vi "ecg_ncs_v2.vi"() -> ()   [LabVIEW 2016]
uses:
  <instrlib>/niUSRP/niUSRP Timestamp.ctl
  C:/Program Files/National Instruments/LabVIEW 2016/examples/Instrument IO/Serial/support/Serial - Settings.ctl
  State.ctl
  <vilib>/Instr/_visa.llb/VISA Configure Serial Port (Instr).vi
  <instrlib>/niUSRP/niUSRP Write Tx Data (2D CDB).vi
  <instrlib>/niUSRP/niUSRP Fetch Rx Data (2D CDB).vi
panel:
  out "ECGsample":i16
  out "PhNcs":dbl
  out "AmpNcs":dbl
  out "AmpNcsDS":dbl
  out "PhNcsDS":dbl
  in  "File Name":string="Test"
  in  "Path":path=path "D:/Research/SummerFall17Spring18/CnC/NCS/EcgNcsCorrelation/Labview Codes/ECG_NCS"
  out "error IO 2":errorcluster={"status"=FALSE, "code"=-1074118647, "source"=""}
  in  "Serial Settings":T1={"baud rate"=57600, "data bits"=8, "parity"=enum."None", "stop bits"=10, "flow control"=0} {"flow control" items=["None"=0, "XON/XOFF"=1, "RTS/CTS"=2, "DTR/DSR"=4]; "stop bits" items=["1.0"=10, "1.5"=15, "2.0"=20]; "data bits" min=5 max=8 step=1; "baud rate" items=["75"=75, "110"=110, "134"=134, "150"=150, "300"=300, "600"=600, "1200"=1200, "1800"=1800, "2400"=2400, "4800"=4800, "7200"=7200, "9600"=9600, "14400"=14400, "19200"=19200, "28800"=28800, "38400"=38400, "56000"=56000, "57600"=57600, "115200"=115200, "128000"=128000, "230400"=230400]}
  in  "VISA resource name":refnum<visa-resource-name>="bmd101"
  out "Packets Recieved":i32
  out "ECG":i16(graph)
  in  "byte count":u32=1
  out "Coerced Rx IQ Rate":dbl
  in  "Sampling Rate":i32=500
  out "Gain":dbl=-15.0
  out "Bandwidth":dbl=56000000.0
  out "Coerced Carrier Frequency":dbl=2000000000.0 format="%#.17g"
  out "Coerced Tx IQ rate":dbl=1000000.0
  out "error IO":errorcluster={"status"=FALSE, "code"=-1074118647, "source"=""}
  in  "Rx Number of Samples":i32=20000
  in  "Tab Control 2":enum32{"NI-294x/295x", "NI-2900/2901"}(tab)=enum."NI-2900/2901"
  in  "Rx carrier frequency [Hz]":dbl=2000000000.0 format="%#_6p"
  in  "Tx carrier frequency [Hz]":dbl=1000000000.0 format="%#_6p"
  in  "Start Trigger Time":T2={"whole seconds"=1, "fractional seconds"=0.0}
  in  "Tab Control":T3(tab)
  out "NCS tag Amp":dbl[](graph)=[0.011967714738528729, 0.012021355192189592, 0.012015275039596582, 0.011969166030167903, 0.011958890166168242, 0.012007893820858737, 0.012022893722444085, 0.011978222225113794, 0.011969989939463181, 0.012003099640895068]
  out "NCS tag Phase":dbl[](graph)=[0.011967714738528729, 0.012021355192189592, 0.012015275039596582, 0.011969166030167903, 0.011958890166168242, 0.012007893820858737, 0.012022893722444085, 0.011978222225113794, 0.011969989939463181, 0.012003099640895068]
  out "Tag Amp":dbl[](graph)
  out "Tag Phase":dbl[](graph)
  out "Tx Waveform Graph":waveform(dbl)[](graph)
  in  "Stop":bool
  in  "Channel 0\nTone Amplitude":dbl=0.707 step=0.05 format="%#.6g"
  in  "Channel 0 \nTone Frequency":dbl=5000.0 format="%#_6p"
  in  "Tx Waveform Size":dbl=2000.0
  in  "Device Name":refnum<k15>="MyB200"
  in  "Tx Gain":dbl=28.0 format="%#_6f"
  in  "Tx IQ Rate":dbl=1000000.0 format="%#_6p"
  in  "Rx Gain":dbl=32.0 format="%#_6f"
  in  "Rx IQ Rate":dbl=1000000.0 format="%#_6p"
  # "Rx Settings"
  # "Tx Settings"
  # "Note that on the NI-2900 and NI-2901, both Rx channels share an LO and both Tx channels share an LO. However, on the NI-294x/295x devices, Rx and Tx of channel 0 share an LO and Rx and Tx of channel 1 share an LO."
  # "Rx: Number of samples should be 1e6/512 in one loop."
  # "This Tx graph should always have end and start tied up since this is being sent in a loop continuously. Otherwise phase jumps will be noticed."
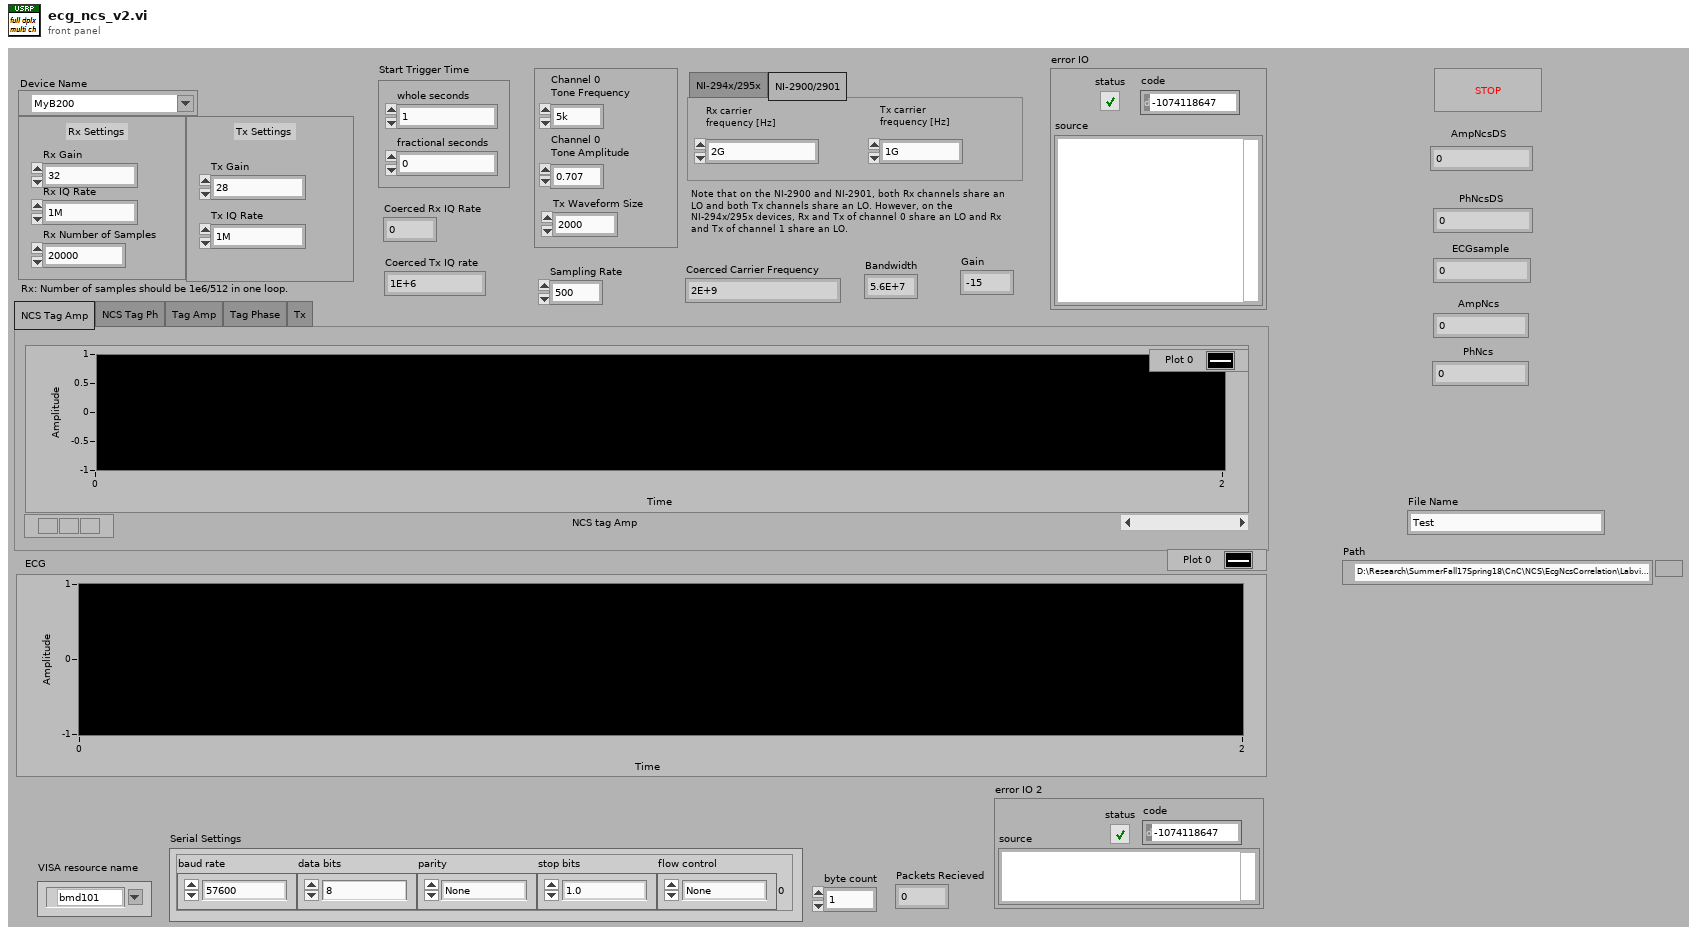
[diagram p1: front panel]
types:
  T1 = typedef "Serial - Settings.ctl" = cluster{"baud rate":u32, "data bits":u16, "parity":enum16{"None", "Odd", "Even", "Mark", "Space"}, "stop bits":u16, "flow control":u16}
  T2 = typedef "niUSRP Timestamp.ctl" = cluster{"whole seconds":u64, "fractional seconds":dbl}
  T3 = enum32{"NCS Tag Amp", "NCS Tag Ph", "Tag Amp", "Tag Phase", "Tx"}
  T4 = typedef "State.ctl" = enum16{"Initialize", "get byte", "check", "packet received", "packet approved"}
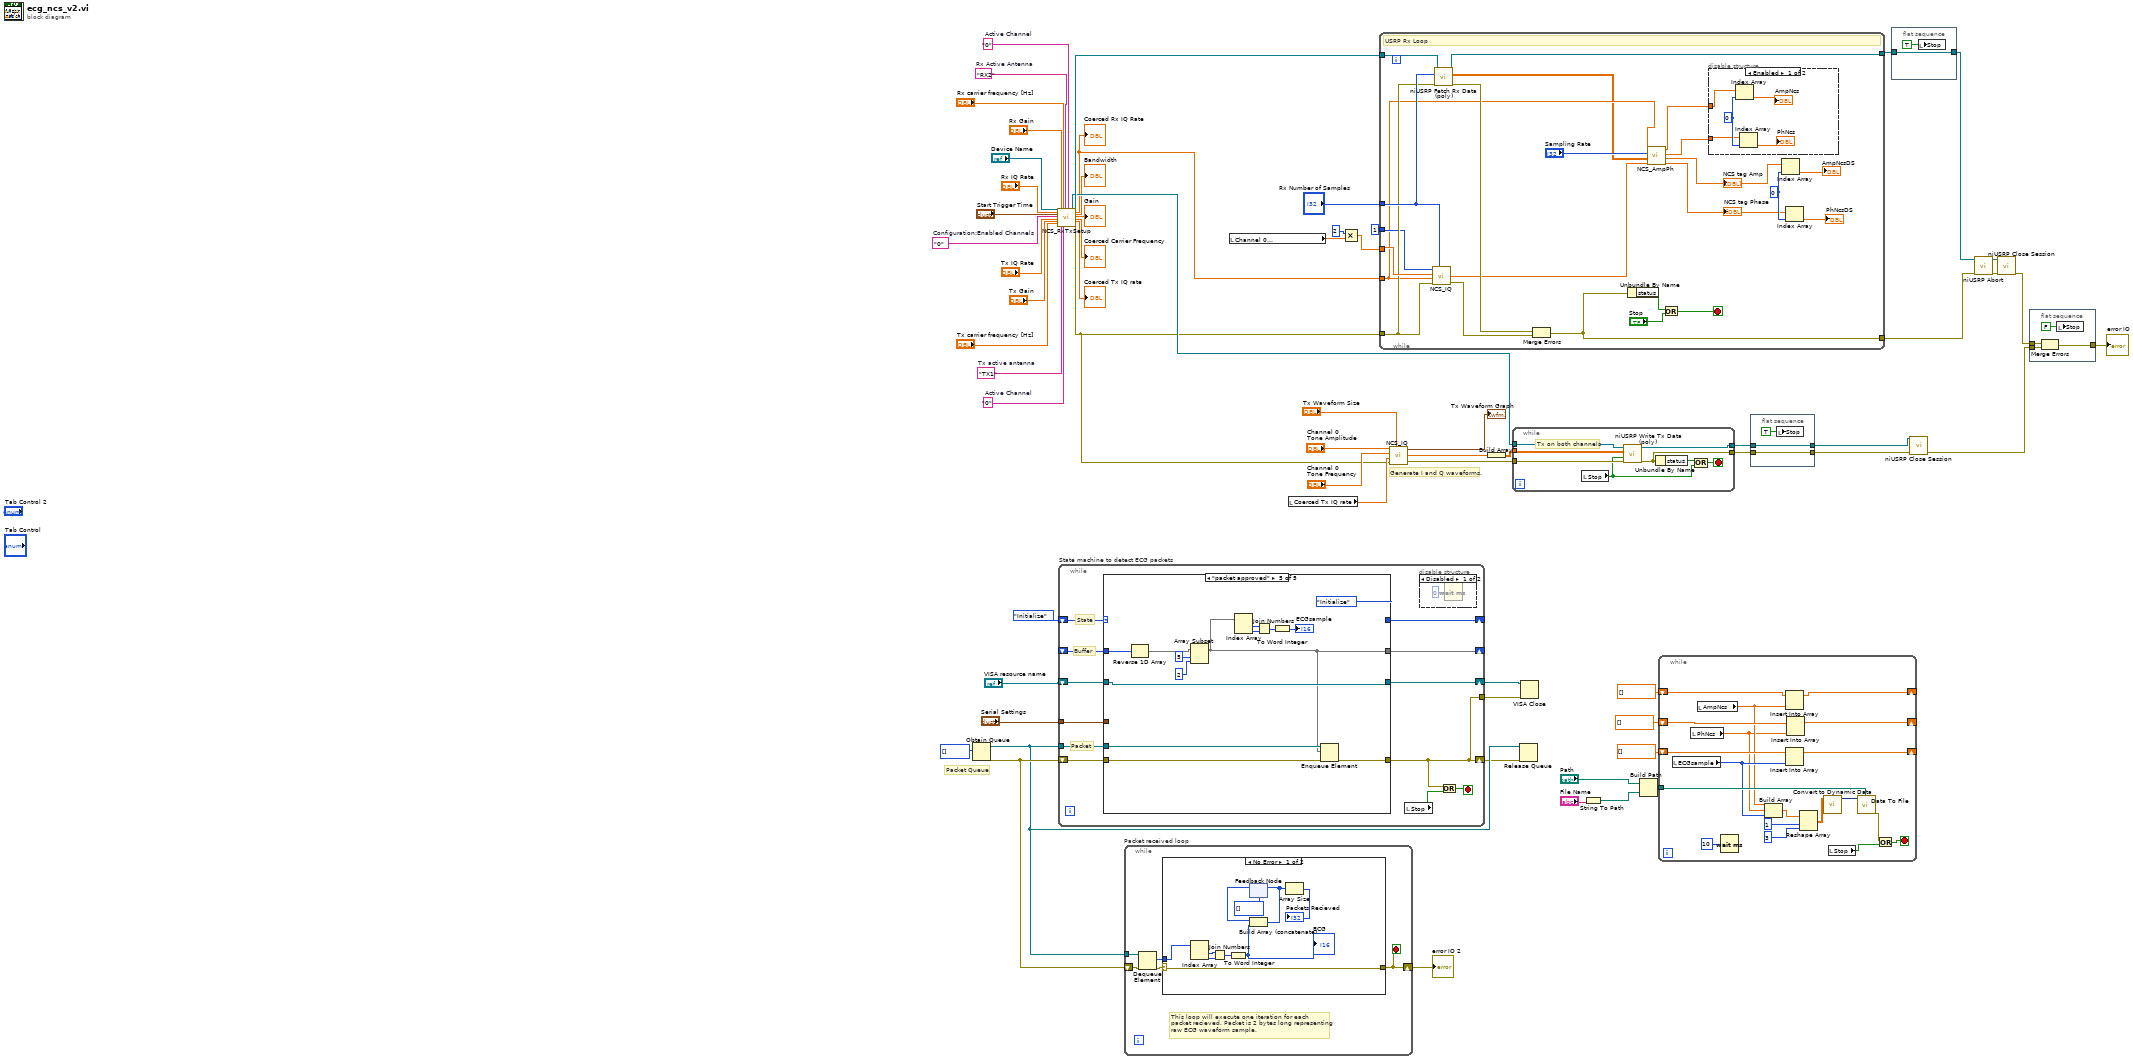
[diagram p0: block diagram]
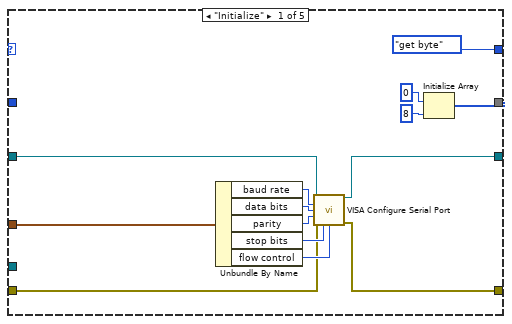
[diagram p4: hidden frame]
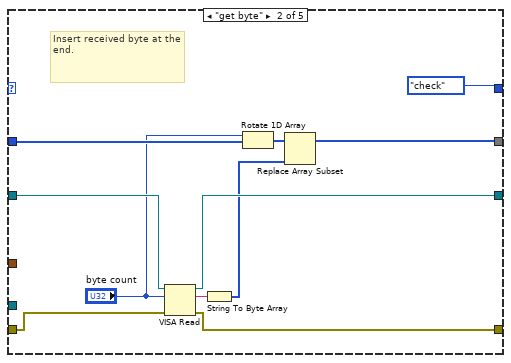
[diagram p5: hidden frame]
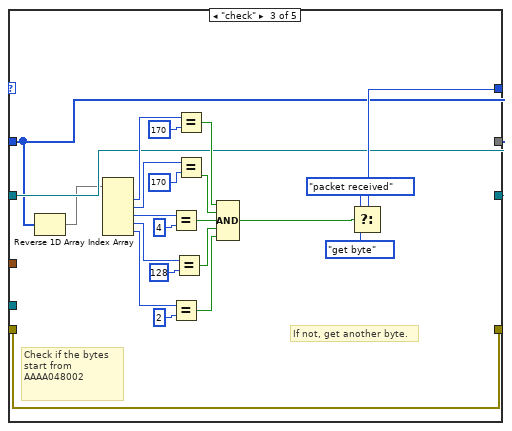
[diagram p6: hidden frame]
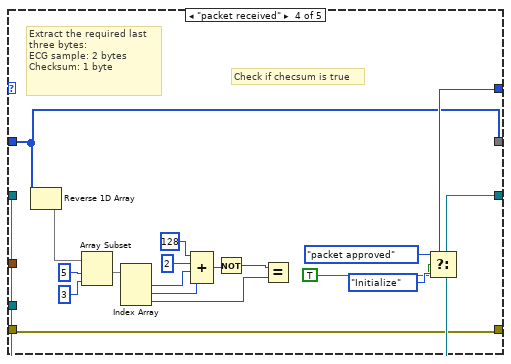
[diagram p7: hidden frame]
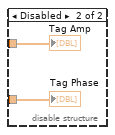
[diagram p8: hidden frame]
diagram:
  w19 = "0"  # Active Channel
  w20 = "0"  # Active Channel
  w55 = "RX2"  # Rx Active Antenna
  w51 = "TX1"  # Tx active antenna
  w37 = "0"  # Configuration:Enabled Channels
  # "Packet Queue"
  # "Generate I and Q waveforms."
  n1 = Obtain Queue(element data type=u8[] []) -> (queue out=w14:refnum<queue>, error out=w15:errorcluster)  [unwired: 4 in, 1 out]
  n2 = call "NCS_RxTxSetup.vi"("IVI Refnum in"="Device Name", "Rx IQ Rate"="Rx IQ Rate", "Start Trigger Time"="Start Trigger Time", "Configuration:Enabled Channels"=w37, "Tx IQ Rate"="Tx IQ Rate", "Tx Gain"="Tx Gain", "Tx carrier frequency [Hz]"="Tx carrier frequency [Hz]", "Rx Gain"="Rx Gain", "Tx active antenna"=w51, "Rx carrier frequency [Hz]"="Rx carrier frequency [Hz]", "Active Channel"=w19, "Rx Active Antenna"=w55, "Active Channel 2"=w20) -> ("session handle out"=w62:refnum<k15>, "IVI Refnum out"=w63:refnum<k15>, "Coerced Rx IQ Rate"=w18:dbl, "Bandwidth"=→"Bandwidth":dbl, "Gain"=→"Gain":dbl, "Carrier Frequency"=→"Coerced Carrier Frequency":dbl, "IQ Rate 2"=→"Coerced Tx IQ rate":dbl, "error out"=w30:errorcluster)  [unwired: 7 in]
  "Coerced Rx IQ Rate" <- w18
  n3 = while "State machine to detect ECG packets" {
    shift-right: [w66] -> w9
    shift-left: w15 -> [w72]
    shift-right: [w75] -> _
    shift-left: State."Initialize" ("State") -> [w74]
    shift-right: [w71] -> _
    shift-left: _ -> [w73]
    tunnel: w14 -> [w70]
    shift-right: [w69] -> w10
    shift-left: "VISA resource name" -> [w68]
    tunnel: "Serial Settings" -> [w67]
    tunnel: [w66] -> w8
    stop <- w65 stop-if-true
    # "State"
    # "Buffer"
    # "Packet"
    n4 = case shown="\"packet approved\"" w74 {
      tunnel: [w87 w99 w103 w126 w144] -> w71
      tunnel: [State."get byte" ("State") State."check" ("f") w123 w132 State."Initialize" ("State")] -> w75
      tunnel: w73 -> [_ w92 w103 w126 w149]
      tunnel: w72 -> [w81 w96 w124 w133 w152]
      tunnel: [w80 w95 w124 w133 w151] -> w66
      tunnel: w70 -> [_ _ _ _ w153]
      tunnel: [w79 w97 w104 w140 w150] -> w69
      tunnel: w68 -> [w78 w98 w104 w140 w150]
      tunnel: w67 -> [w77 _ _ _ _]
      frame "Initialize" {
        n5 = Unbundle By Name(w77) -> ("baud rate"=w86:u32, "data bits"=w85:u16, "parity"=w84:enum16{"None", "Odd", "Even", "Mark", "Space"}, "stop bits"=w83:u16, "flow control"=w82:u16)
        n6 = call-poly "VISA Configure Serial Port"("VISA resource name"=w78, "baud rate (9600)"=w86, "data bits (8)"=w85, "parity (0:none)"=w84, "error in (no error)"=w81, "stop bits (10: 1 bit)"=w83, "flow control (0:none)"=w82) -> ("VISA resource name out"=w79:refnum<visa-resource-name>, "error out"=w80:errorcluster)  [unwired: 3 in, 4 out]
        n7 = Initialize Array(u8 0, 8 ("dimension size")) -> (w87:u8[])
      }
      frame "get byte" {
        # "Insert received byte at the end."
        n8 = VISA Read(VISA resource name=w98, byte count="byte count", error in (no error)=w96) -> (VISA resource name out=w97:refnum<visa-resource-name>, read buffer=w94:string, error out=w95:errorcluster)  [unwired: 1 out]
        n9 = String To Byte Array(string=w94) -> (unsigned byte array=w93:u8[])
        n10 = Rotate 1D Array(1:w92, 2:"byte count") -> (0:w100:u8[])
        n11 = Replace Array Subset(array=w100, new element=w93) -> (w99:u8[])  [unwired: 1 in]
      }
      frame "check" {
        # "If not, get another byte."
        # "Check if the bytes start from AAAA048002"
        n12 = Reverse 1D Array(array=w103) -> (reversed array=w102:u8[])
        n13 = Index Array(array=w102) -> (element #1=w110:u8, element #2=w109:u8, element #3=w108:u8, element #4=w107:u8, element #5=w106:u8)  [unwired: 5 in]
        n14 = Equal?(x=w108, y=u8 4 ("element")) -> (x = y?=w113:bool)
        n15 = Equal?(x=w106, y=u8 2 ("element")) -> (x = y?=w111:bool)
        n16 = Equal?(x=w107, y=u8 128 ("element")) -> (x = y?=w112:bool)
        n17 = Equal?(x=w110, y=u8 170 ("element")) -> (x = y?=w115:bool)
        n18 = Equal?(x=w109, y=u8 170 ("element")) -> (x = y?=w114:bool)
        n19 = Compound Arithmetic op=AND(w115, w114, w113, w112, w111) -> (w105:bool)
        n20 = Select(t=State."packet received" ("f"), s=w105, f=State."get byte") -> (s? t:f=w123:T4)
      }
      frame "packet received" {
        # "Check if checsum is true"
        # "Extract the required last three bytes: \nECG sample: 2 bytes\nChecksum: 1 byte"
        n21 = Reverse 1D Array(array=w126) -> (reversed array=w125:u8[])
        n22 = Array Subset(array=w125, index=5, length=3 ("index")) -> (w139:u8[])
        n23 = Index Array(array=w139) -> (element #1=w134:u8, element #2=w135:u8, element #3=w136:u8)  [unwired: 3 in]
        n24 = Compound Arithmetic op=ADD(u8 128 ("element"), u8 2 ("element"), w134, w135) -> (w129:u8)
        n25 = Not(x=w129) -> (.not. x?=w128:u8)
        n26 = Equal?(x=w128, y=w136) -> ()  [unwired: 1 out]
        n27 = Select(t=State."packet approved" ("State"), s=TRUE, f=State."Initialize" ("State")) -> (s? t:f=w132:T4)
      }
      frame "packet approved" {
        n28 = Reverse 1D Array(array=w149) -> (reversed array=w148:u8[])
        n29 = Array Subset(array=w148, index=5, length=2 ("index")) -> (w144:u8[])
        n30 = Index Array(array=w144) -> (element #1=w143:u8, element #2=w146:u8)  [unwired: 2 in]
        n31 = Join Numbers(hi=w143, lo=w146) -> ((hi.lo)=w147:u16)
        n32 = To Word Integer(number=w147) -> (16bit integer=→"ECGsample":i16)
        n33 = Enqueue Element(queue=w153, element=w144, error in (no error)=w152) -> (error out=w151:errorcluster)  [unwired: 1 in, 2 out]
      }
    }
    n34 = local read "Stop"() -> (w64:bool)
    n35 = disable-structure shown="Disabled" {
      frame Disabled {
        n36 = Wait (ms)(milliseconds to wait=u32 0) -> ()  [unwired: 1 out]
      }
      frame Enabled {
      }
    }
    n37 = Or(x=w66, y=w64) -> (x .or. y?=w65:bool)
  }
  n38 = while "Packet received loop" {
    shift-right: [w157] -> w11
    shift-left: w15 -> [w161]
    tunnel: w14 -> [w160]
    stop <- w157 stop-if-true
    # "This loop will execute one iteration for each\npacket recieved. Packet is 2 bytes long representing \nraw ECG waveform sample."
    n39 = Dequeue Element(queue=w160, error in (no error)=w161) -> (element=w159:u8[], error out=w158:errorcluster)  [unwired: 1 in, 2 out]
    n40 = case shown="No Error" w158 {
      selector: w158 -> [w171 w172]
      tunnel: w159 -> [w170 _]
      tunnel: [w171 w172] -> w157
      frame No Error {
        n41 = Index Array(array=w170) -> (element #1=w169:u8, element #2=w168:u8)  [unwired: 2 in]
        n42 = Join Numbers(hi=w169, lo=w168) -> ((hi.lo)=w167:u16)
        n43 = To Word Integer(number=w167) -> (16bit integer=w162:i16)
        "ECG" <- w162
        n44 = feedback #1(i32[] []) -> (w165:i32[])
        n45 = Build Array (concatenate)(w165, w162) -> (w164:i32[])
        n46 = feedback-in #1(w164) -> ()
        n47 = Array Size(array=w164) -> (size(s)=→"Packets Recieved":i32)
      }
      frame Error {
      }
    }
  }
  "error IO 2" <- w11
  n48 = local read "Channel 0 \nTone Frequency"() -> (w36:dbl)
  n49 = local read "Coerced Tx IQ rate"() -> (w31:dbl)
  n50 = Multiply(x=2, y=w36) -> (x*y=w35:dbl)
  n51 = while {
    tunnel: w63 -> [w195]
    tunnel: w30 -> [w188]
    tunnel: [w194] -> w47
    tunnel: "Rx Number of Samples" -> [w190]
    tunnel: w18 -> [w184]
    tunnel: [w185] -> w39
    tunnel: w35 -> [w189]
    tunnel: 1 -> [w186]
    stop <- w191 stop-if-true
    w176 = 0
    # "USRP Rx Loop"
    n52 = call "NCS_IQ.vi"("Tone Amplitude"=w186, "Waveform Size"=w190, "Tone Frequency"=w189, "Coerced IQ rate"=w184, "error in (no error)"=w188) -> ("IQ waveform array"=w181:cdb[], "error out"=w187:errorcluster)  [unwired: 1 in, 1 out]
    n53 = call-poly <instrlib>:"niUSRP Fetch Rx Data (poly).vi"("session handle"=w195, "number of samples"=w190, "error in (no error)"=w188) -> ("session handle out"=w194:refnum<k15>, "data"=w182:cdb[][], "error out"=w192:errorcluster)  [unwired: 9 in, 1 out]
    n54 = Merge Errors(w192, w187) -> (w185:errorcluster)
    n55 = Unbundle By Name(w185) -> ("status"=w193:bool)
    n56 = call "NCS_AmpPh.vi"("IQ"=w181, "data"=w182, "Sampling Rate"="Sampling Rate", "Coerced Rx IQ Rate"=w184) -> ("Phase DownSampled"=w175:dbl[], "Amp DownSampled"=w177:dbl[], "Phase"=w179:dbl[], "Amplitude"=w180:dbl[])  [unwired: 4 in]
    "NCS tag Amp" <- w177
    "NCS tag Phase" <- w175
    n57 = Or(x=w193, y="Stop") -> (x .or. y?=w191:bool)
    n58 = disable-structure shown="Enabled" {
      disable-tunnel: w180 -> [w199 w202]
      disable-tunnel: w179 -> [w198 w201]
      frame Enabled {
        w200 = 0
        n59 = Index Array(array=w199, index=w200) -> (element=→"AmpNcs":dbl)
        n60 = Index Array(array=w198, index=w200) -> (element=→"PhNcs":dbl)
      }
      frame Disabled {
        "Tag Amp" <- w202
        "Tag Phase" <- w201
      }
    }
    n61 = Index Array(array=w177, index=w176) -> (element=→"AmpNcsDS":dbl)
    n62 = Index Array(array=w175, index=w176) -> (element=→"PhNcsDS":dbl)
  }
  n63 = call "NCS_IQ.vi"("Tone Amplitude"="Channel 0\nTone Amplitude", "Waveform Size"="Tx Waveform Size", "Tone Frequency"="Channel 0 \nTone Frequency", "Coerced IQ rate"=w31, "error in (no error)"=w30) -> ("IQ waveform"=→"Tx Waveform Graph":waveform(dbl)[], "IQ waveform array"=w28:cdb[], "error out"=w29:errorcluster)  [unwired: 1 in]
  n64 = Build Array(w28) -> (w59:cdb[][])
  n65 = while {
    tunnel: w62 -> [w210]
    tunnel: w29 -> [w209]
    tunnel: [w207] -> w50
    tunnel: [w205] -> w45
    tunnel: w59 -> [w203]
    stop <- w206 stop-if-true
    # "Tx on both channels"
    n66 = local read "Stop"() -> (w204:bool)
    n67 = call-poly <instrlib>:"niUSRP Write Tx Data (poly).vi"("session handle"=w210, "data"=w203, "end of data?"=w204, "error in (no error)"=w209) -> ("session handle out"=w205:refnum<k15>, "error out"=w207:errorcluster)  [unwired: 10 in]
    n68 = Unbundle By Name(w207) -> ("status"=w208:bool)
    n69 = Compound Arithmetic op=OR(w208, w204) -> (w206:bool)
  }
  n70 = Release Queue(queue=w14, error in (no error)=w9) -> ()  [unwired: 1 in, 3 out]
  n71 = VISA Close(VISA resource name=w10, error in (no error)=w8) -> ()  [unwired: 1 out]
  n72 = String To Path(string="File Name") -> (path=w6:path)
  n73 = Build Path(base path="Path", name or relative path=w6) -> (appended path=w2:path)
  n74 = while {
    shift-right: [w224] -> _
    shift-left: dbl[] [] -> [w221]
    shift-right: [w223] -> _
    shift-left: dbl[] [] -> [w220]
    tunnel: w2 -> [w222]
    shift-right: [w213] -> _
    shift-left: dbl[] [] -> [w214]
    stop <- w227 stop-if-true
    n75 = local read "ECGsample"() -> (w219:i16)
    n76 = local read "PhNcs"() -> (w211:dbl)
    n77 = local read "AmpNcs"() -> (w212:dbl)
    n78 = Wait (ms)(milliseconds to wait=u32 10) -> ()  [unwired: 1 out]
    n79 = Build Array(w212, w211, w219) -> (w218:dbl[])
    n80 = Insert Into Array(array=w214, new element=w212) -> (w213:dbl[])  [unwired: 1 in]
    n81 = Insert Into Array(array=w220, new element=w219) -> (w223:dbl[])  [unwired: 1 in]
    n82 = Insert Into Array(array=w221, new element=w211) -> (w224:dbl[])  [unwired: 1 in]
    n83 = Reshape Array(w218, 1 ("dimension size"), 3 ("dimension size")) -> (w215:dbl[][])
    n84 = call "Convert to Dynamic Data"("2D Array"=w215) -> ("Dynamic Data Type"=w228:dynamicdata)  [unwired: 3 in]
    n85 = local read "Stop"() -> (w225:bool)
    n86 = call "Data To File"("Signals"=w228, "Filename"=w222) -> ("error out"=w226:errorcluster)  [unwired: 15 in, 2 out]
    n87 = Or(x=w226, y=w225) -> (x .or. y?=w227:bool)
  }
  n88 = flat-sequence {
    tunnel: [w231] -> w49
    tunnel: w50 -> [w231]
    tunnel: [w230] -> w46
    tunnel: w45 -> [w230]
    frame #0 {
      n89 = local write "Stop"(TRUE ("STOP")) -> ()
    }
  }
  n90 = flat-sequence {
    tunnel: [w233] -> w48
    tunnel: w47 -> [w233]
    frame #0 {
      n91 = local write "Stop"(TRUE ("STOP")) -> ()
    }
  }
  n92 = call <instrlib>:"niUSRP Close Session.vi"("session handle"=w46, "error in (no error)"=w49) -> ("error out"=w44:errorcluster)  [unwired: 13 in]
  n93 = call <instrlib>:"niUSRP Abort.vi"("session handle"=w48, "error in (no error)"=w39) -> ("session handle out"=w61:refnum<k15>, "error out"=w60:errorcluster)  [unwired: 12 in]
  n94 = call <instrlib>:"niUSRP Close Session.vi"("session handle"=w61, "error in (no error)"=w60) -> ("error out"=w41:errorcluster)  [unwired: 13 in]
  n95 = flat-sequence {
    tunnel: w44 -> [w237]
    tunnel: [w236] -> w42
    tunnel: w41 -> [w235]
    frame #0 {
      n96 = Merge Errors(w235, w237) -> (w236:errorcluster)
      n97 = local write "Stop"(FALSE ("STOP")) -> ()
    }
  }
  "error IO" <- w42
